vi "FMDemod (SubVI).vi"(10 "QSamples":dbl[](array[numeric]), 11 "ISamples":dbl[](array[numeric])) -> (3 "Baseband":dbl[](array[numeric]))   [LabVIEW 2013]
uses:
  FMDemodRTLSDR_NET/for_redistribution_files_only/FMDemodRTLSDR_NET.dll
panel:
  out "size(s)":i32
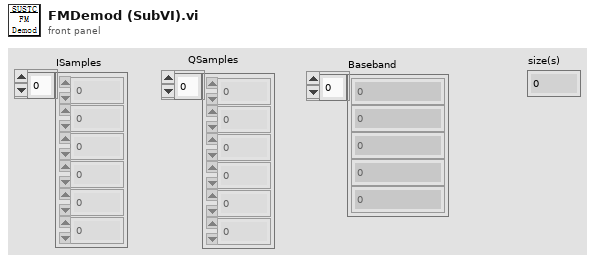
[diagram p1: front panel]
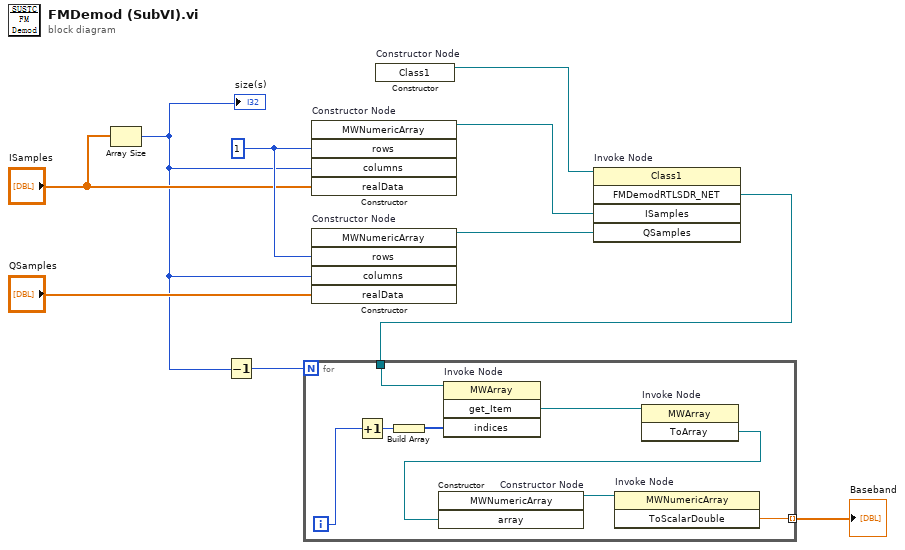
[diagram p0: block diagram]
diagram:
  w6 = 1 ("rows")
  n1 = Array Size(array="ISamples") -> (size(s)=w4:i32)
  "size(s)" <- w4
  n2 = Decrement(x=w4) -> (x-1=w1:i32)
  n3 = constructor on="Constructor Node" class="MWNumericArray"("rows"=w6, "columns"=w4, "realData"="ISamples") -> (reference out=w8:refnum<k24>)  [unwired: 3 in, 5 out]
  n4 = constructor on="Constructor Node" class="MWNumericArray"("rows"=w6, "columns"=w4, "realData"="QSamples") -> (reference out=w7:refnum<k24>)  [unwired: 3 in, 5 out]
  n5 = constructor on="Constructor Node" class="Class1"() -> (reference out=w9:refnum<k24>)  [unwired: 3 in, 2 out]
  n6 = invoke on="Invoke Node" class="Class1" method="FMDemodRTLSDR_NET"(reference=w9, "ISamples"=w8, "QSamples"=w7) -> ("FMDemodRTLSDR_NET"=w2:refnum<k24>)  [unwired: 2 in, 4 out]
  n7 = for {
    N: w1 -> [_]
    tunnel: w2 -> [w13]
    tunnel: [w11] -> w3 mode=indexing
    i -> [w18]
    n8 = Increment(x=w18) -> (x+1=w17:i32)
    n9 = Build Array(w17) -> (w16:i32[])
    n10 = invoke on="Invoke Node" class="MWArray" method="get_Item"(reference=w13, "indices"=w16) -> ("get_Item"=w15:refnum<k24>)  [unwired: 2 in, 3 out]
    n11 = invoke on="Invoke Node" class="MWArray" method="ToArray"(reference=w15) -> ("ToArray"=w12:refnum<k24>)  [unwired: 2 in, 2 out]
    n12 = constructor on="Constructor Node" class="MWNumericArray"("array"=w12) -> (reference out=w14:refnum<k24>)  [unwired: 3 in, 3 out]
    n13 = invoke on="Invoke Node" class="MWNumericArray" method="ToScalarDouble"(reference=w14) -> ("ToScalarDouble"=w11:dbl)  [unwired: 2 in, 2 out]
  }
  "Baseband" <- w3
